vi "isInitialized.vi"(6 "Delay between send and receive [ms]":i32=100, 8 "error in (no error)":errorcluster, 11 "Monochromator in":refnum<class "Monochromator.lvclass">) -> (0 "error out":errorcluster, 2 "mono is initialized?":bool, 3 "Monochromator out":refnum<class "Monochromator.lvclass">)   [LabVIEW 2020, in "horiba.lvlib" / "Monochromator.lvclass"]
doc: "This command returns true when the mono is initialized. Otherwise it returns false.\n\nNote: This command may also return false when the mono is busy with another command."
uses:
  Monochromator.lvclass
  Monochromator.lvclass/Monochromator.ctl
  d9b87029-586e-44ee-a6e5-d4a5e0edce38.vi
  b59fd1e7-dcda-425c-bd6c-61aafb79e7f4.vi
  GenericDevice/GenericDevice.lvclass
  IsInitialized.ctl
  <vilib>/JDP Science/JSONtext/JSONtext.lvlib
panel:
  # "Connector Pane"
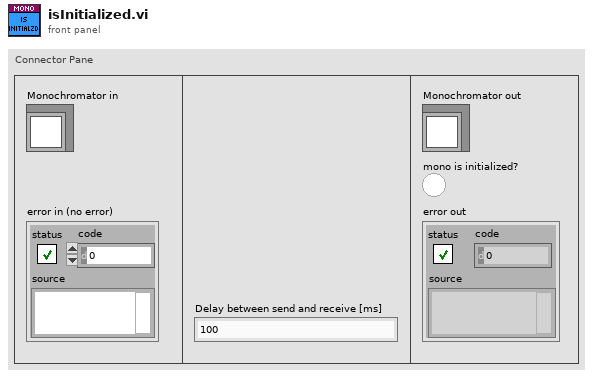
[diagram p1: front panel]
types:
  T1 = typedef "horiba.lvlib/Monochromator.lvclass/IsInitialized.ctl" = cluster{"initialized":bool}
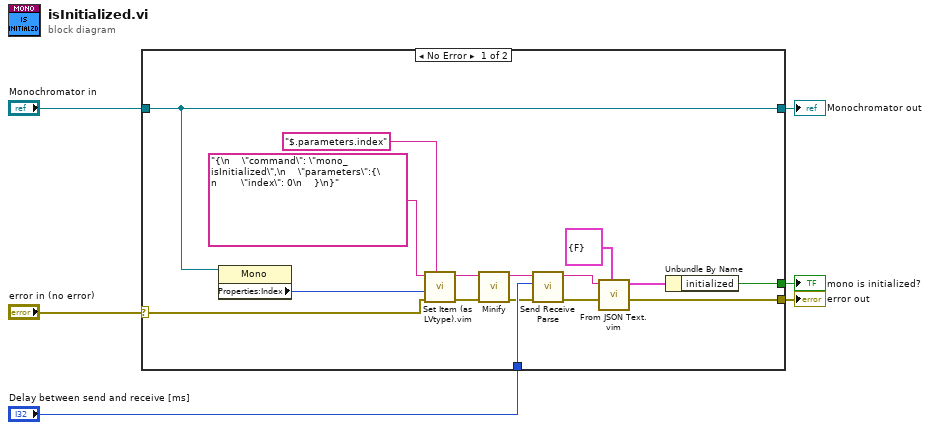
[diagram p0: block diagram]
diagram:
  n1 = case shown="No Error" "error in (no error)" {
    selector: "error in (no error)" -> [w18 w24]
    tunnel: [w17 w24] -> w5
    tunnel: [w20 w23] -> w3
    tunnel: "Monochromator in" -> [w20 w23]
    tunnel: [w12 _] -> w2
    tunnel: "Delay between send and receive [ms]" -> [w11 _]
    frame No Error {
      n2 = property class="Mono"(reference=w20) -> ("Properties:Index"=w19:i32)  [unwired: 1 in, 2 out]
      n3 = call "Set Item (as LVtype).vim"("$Path or Item Name"="$.parameters.index", "error in (no error)"=w18, "Anything"=w19, "JSON"="{\n    \"command\": \"mono_isInitialized\",\n    \"parameters\":{\n        \"index\": 0\n    }\n}") -> ("error out"=w16:errorcluster, "<JSON>"=w8:string)  [unwired: 4 in, 1 out]
      n4 = call <vilib>:"Minify.vi"("error in (no error)"=w16, "JSON"=w8) -> ("error out"=w9:errorcluster, "<JSON>"=w7:string)  [unwired: 7 in, 1 out]
      n5 = call "Send Receive Parse.vi"("error in"=w9, "Delay between send and receive [ms]"=w11, "<JSON>"=w7) -> ("error out"=w14:errorcluster, "results-JSON string"=w15:string)  [unwired: 6 in, 1 out]
      n6 = call "From JSON Text.vim"("Data Type and Default Value"=T1 {"initialized"=FALSE} ("Mono is initialized?"), "error in (no error)"=w14, "JSON"=w15) -> ("error out"=w17:errorcluster, "Data out"=w13:T1)  [unwired: 7 in]
      n7 = Unbundle By Name(w13) -> ("initialized"=w12:bool)
    }
    frame Error {
    }
  }
  "error out" <- w5
  "Monochromator out" <- w3
  "mono is initialized?" <- w2
